vi "resonanc_sim.vi"(8 "sim params":T1, 11 "X":dbl) -> (1 "noise estimate":dbl, 2 "sim. y":dbl, 3 "X copy":dbl)   [LabVIEW 2015]
uses:
  <vilib>/Analysis/NI_AALBase.lvlib
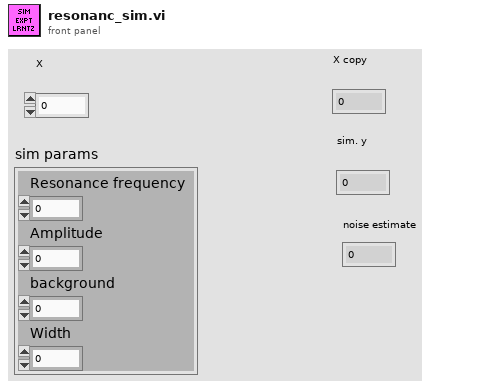
[diagram p1: front panel]
types:
  T1 = cluster{"Resonance frequency":dbl, "Amplitude":dbl, "background":dbl, "Width":dbl}
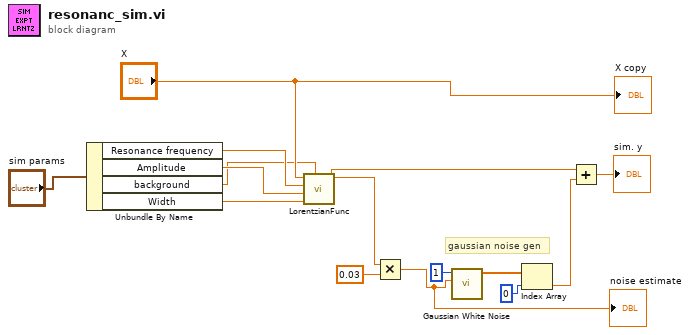
[diagram p0: block diagram]
diagram:
  # "gaussian noise gen"
  n1 = Unbundle By Name("sim params") -> ("Resonance frequency"=w7:dbl, "Amplitude"=w6:dbl, "background"=w5:dbl, "Width"=w4:dbl)
  n2 = call "LorentzianFunc.vi"("B"=w5, "d"=w4, "A"=w6, "x0"=w7, "X"="X") -> ("B+A/[1+(X-X0)^2 / d^2]"=w2:dbl)  [unwired: 6 in]
  n3 = Multiply(x=w2, y=0.03) -> (x*y=w1:dbl)
  "noise estimate" <- w1
  n4 = call <vilib>:"Gaussian White Noise.vi"("standard deviation"=w1, "samples"=1) -> ("Gaussian noise pattern"=w11:dbl[])  [unwired: 8 in, 1 out]
  n5 = Index Array(array=w11, index=0) -> (element=w10:dbl)
  n6 = Add(x=w2, y=w10) -> (x+y=→"sim. y":dbl)
  "X copy" <- "X"
